vi "FPGAOutput.vi"() -> ()   [LabVIEW 2016]
uses:
  <vilib>/rvi/eio/common/nirviEmuTemplateMethod_errors.vi
  <vilib>/rvi/Emulation/niFpgaGetClockAttributes.vi
  <vilib>/rvi/Emulation/niFpgaSctlEmulationGetInTimedLoop.vi
  <vilib>/rvi/Emulation/niFpgaEmulationReportErrorSimple.vi
  <vilib>/rvi/Emulation/niFpgaCriticalErrorInLSC.vi
  <vilib>/eio/EIONode/EIONode.xnode
panel:
  in  "Both":bool
  in  "Ch1":bool
  in  "Amplitude":fxp<+,32,0>
  in  "Frequency":fxp<+,32,0>=2.491287887096405e-08
  in  "StopButton":bool
  out "State":i16
  in  "Ch0":bool
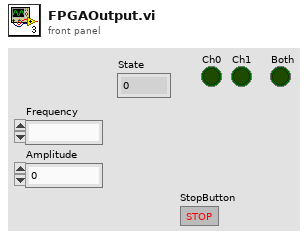
[diagram p1: front panel]
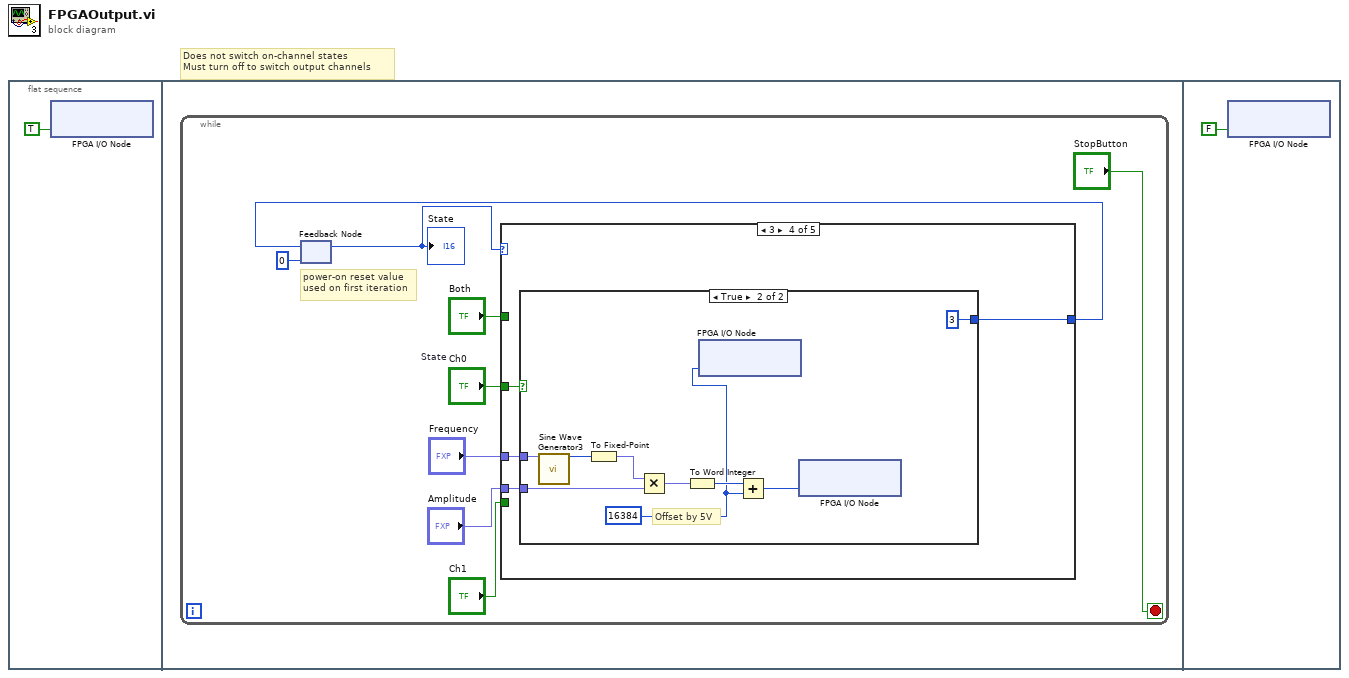
[diagram p0: block diagram]
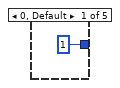
[diagram p2: hidden frame]
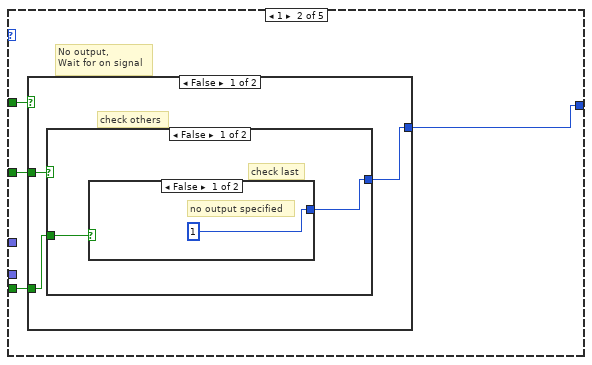
[diagram p3: hidden frame]
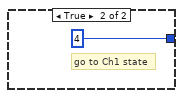
[diagram p4: hidden frame]
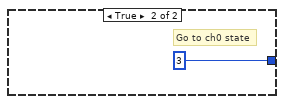
[diagram p5: hidden frame]
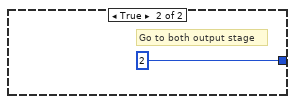
[diagram p6: hidden frame]
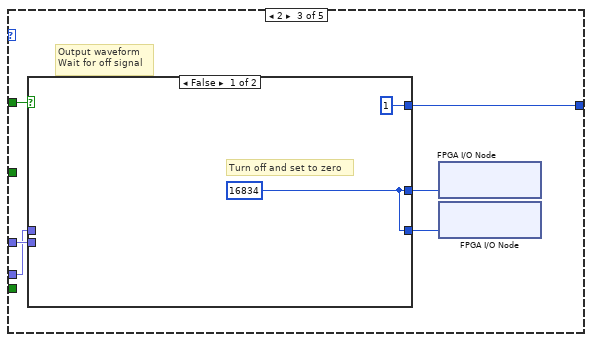
[diagram p7: hidden frame]
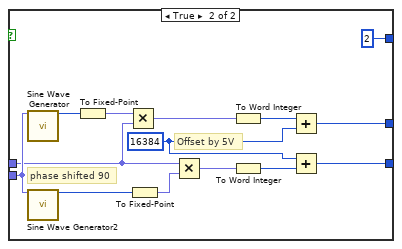
[diagram p8: hidden frame]
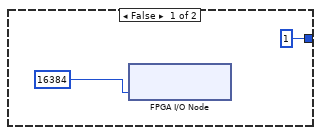
[diagram p9: hidden frame]
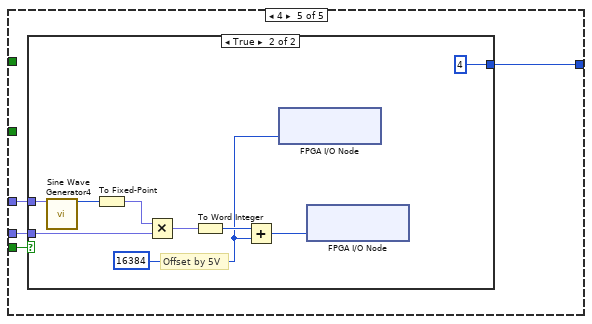
[diagram p10: hidden frame]
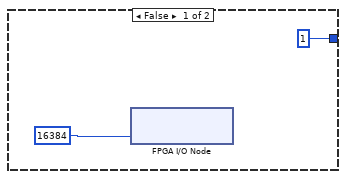
[diagram p11: hidden frame]
diagram:
  # "Does not switch on-channel states\nMust turn off to switch output channels"
  n1 = flat-sequence {
    frame #0 {
      n2 = xnode "FPGA I/O Node"("Mod6/CH0"=TRUE) -> ()  [unwired: 1 in, 1 out]
    }
    frame #1 {
      n3 = while {
        stop <- "StopButton" stop-if-true
        # "power-on reset value\nused on first iteration"
        n4 = feedback #1 "State"(i16 0) -> (w10:i16)
        "State" <- w10
        n5 = case shown="3" w10 {
          tunnel: [i16 1 w15 w30 w49 w65] -> w9
          tunnel: "Both" -> [_ w14 w27 _ _]
          tunnel: "Ch0" -> [_ w13 _ w50 _]
          tunnel: "Ch1" -> [_ w12 _ _ w64]
          tunnel: "Frequency" -> [_ _ w26 w47 w63]
          tunnel: "Amplitude" -> [_ _ w25 w48 w62]
          frame 0, Default {
          }
          frame 1 {
            # "No output,\nWait for on signal"
            n6 = case shown="False" w14 {
              tunnel: [w17 i16 2] -> w15
              tunnel: w13 -> [w18 _]
              tunnel: w12 -> [w16 _]
              frame False {
                # "check others"
                n7 = case shown="False" w18 {
                  tunnel: [w20 i16 3] -> w17
                  tunnel: w16 -> [w19 _]
                  frame False {
                    # "check last"
                    n8 = case shown="False" w19 {
                      tunnel: [i16 1 i16 4] -> w20
                      frame False {
                        # "no output specified"
                      }
                      frame True {
                        # "go to Ch1 state"
                      }
                    }
                  }
                  frame True {
                    # "Go to ch0 state"
                  }
                }
              }
              frame True {
                # "Go to both output stage"
              }
            }
          }
          frame 2 {
            # "Output waveform\nWait for off signal"
            n9 = case shown="False" w27 {
              tunnel: [i16 1 i16 2] -> w30
              tunnel: [w31 w41] -> w29
              tunnel: [w31 w35] -> w28
              tunnel: w26 -> [_ w34]
              tunnel: w25 -> [_ w33]
              frame False {
                w31 = i16 16834
                # "Turn off and set to zero"
              }
              frame True {
                w37 = i16 16384 ("y")
                # "phase shifted 90"
                # "Offset by 5V"
                n10 = call "Sine Wave Generator"("frequency (periods/tick)"=w34) -> ("sine out"=w45:i16)  [unwired: 14 in]
                n11 = call "Sine Wave Generator2"("frequency (periods/tick)"=w34) -> ("sine out"=w40:i16)  [unwired: 14 in]
                n12 = To Fixed-Point(number=w45) -> (fixed-point=w44:fxp<+/-,32,16>)  [unwired: 1 in]
                n13 = Multiply(x=w44, y=w33) -> (x*y=w42:fxp<+/-,64,16>)
                n14 = To Fixed-Point(number=w40) -> (fixed-point=w38:fxp<+/-,32,16>)  [unwired: 1 in]
                n15 = Multiply(x=w33, y=w38) -> (x*y=w39:fxp<+/-,64,16>)
                n16 = To Word Integer(number=w42) -> (16bit integer=w43:i16)
                n17 = To Word Integer(number=w39) -> (16bit integer=w36:i16)
                n18 = Add(x=w43, y=w37) -> (x+y=w41:i16)
                n19 = Add(x=w37, y=w36) -> (x+y=w35:i16)
              }
            }
            n20 = xnode "FPGA I/O Node"("Mod5/AO1"=w29) -> ()  [unwired: 1 in, 1 out]
            n21 = xnode "FPGA I/O Node"("Mod5/AO0"=w28) -> ()  [unwired: 1 in, 1 out]
          }
          frame 3 {
            n22 = case shown="True" w50 {
              tunnel: [i16 1 i16 3] -> w49
              tunnel: w48 -> [_ w55]
              tunnel: w47 -> [_ w54]
              frame False {
                n23 = xnode "FPGA I/O Node"("Mod5/AO0"=i16 16384 ("y")) -> ()  [unwired: 1 in, 1 out]
              }
              frame True {
                w53 = i16 16384 ("y")
                # "Offset by 5V"
                n24 = call "Sine Wave Generator3"("frequency (periods/tick)"=w54) -> ("sine out"=w61:i16)  [unwired: 14 in]
                n25 = To Fixed-Point(number=w61) -> (fixed-point=w60:fxp<+/-,32,16>)  [unwired: 1 in]
                n26 = Multiply(x=w60, y=w55) -> (x*y=w58:fxp<+/-,64,16>)
                n27 = To Word Integer(number=w58) -> (16bit integer=w59:i16)
                n28 = xnode "FPGA I/O Node"("Mod5/AO1"=w53) -> ()  [unwired: 1 in, 1 out]
                n29 = Add(x=w59, y=w53) -> (x+y=w57:i16)
                n30 = xnode "FPGA I/O Node"("Mod5/AO0"=w57) -> ()  [unwired: 1 in, 1 out]
              }
            }
          }
          frame 4 {
            n31 = case shown="True" w64 {
              tunnel: [i16 1 i16 4] -> w65
              tunnel: w62 -> [_ w70]
              tunnel: w63 -> [_ w69]
              frame False {
                n32 = xnode "FPGA I/O Node"("Mod5/AO1"=i16 16384 ("y")) -> ()  [unwired: 1 in, 1 out]
              }
              frame True {
                w68 = i16 16384 ("y")
                # "Offset by 5V"
                n33 = call "Sine Wave Generator4"("frequency (periods/tick)"=w69) -> ("sine out"=w76:i16)  [unwired: 14 in]
                n34 = To Fixed-Point(number=w76) -> (fixed-point=w75:fxp<+/-,32,16>)  [unwired: 1 in]
                n35 = Multiply(x=w75, y=w70) -> (x*y=w73:fxp<+/-,64,16>)
                n36 = To Word Integer(number=w73) -> (16bit integer=w74:i16)
                n37 = Add(x=w74, y=w68) -> (x+y=w72:i16)
                n38 = xnode "FPGA I/O Node"("Mod5/AO0"=w68) -> ()  [unwired: 1 in, 1 out]
                n39 = xnode "FPGA I/O Node"("Mod5/AO1"=w72) -> ()  [unwired: 1 in, 1 out]
              }
            }
          }
        }
        n40 = feedback-in #1(w9) -> ()
      }
    }
    frame #2 {
      n41 = xnode "FPGA I/O Node"("Mod6/CH0"=FALSE) -> ()  [unwired: 1 in, 1 out]
    }
  }
